vi "Send Message.vi"(0 "object in":refnum<class "Laser_Ethernet.lvclass">, 5 "error in (no error)":errorcluster) -> (14 "object out":refnum<class "Laser_Ethernet.lvclass">, 19 "error out":errorcluster)   [LabVIEW 2023, in "Laser_Ethernet.lvclass"]
uses:
  Laser_Ethernet.lvclass
  Laser_Ethernet.lvclass/Laser_Ethernet.ctl
panel:
  in  "Size of Data":u32
  in  "Command":u16
  in  "Data":variant
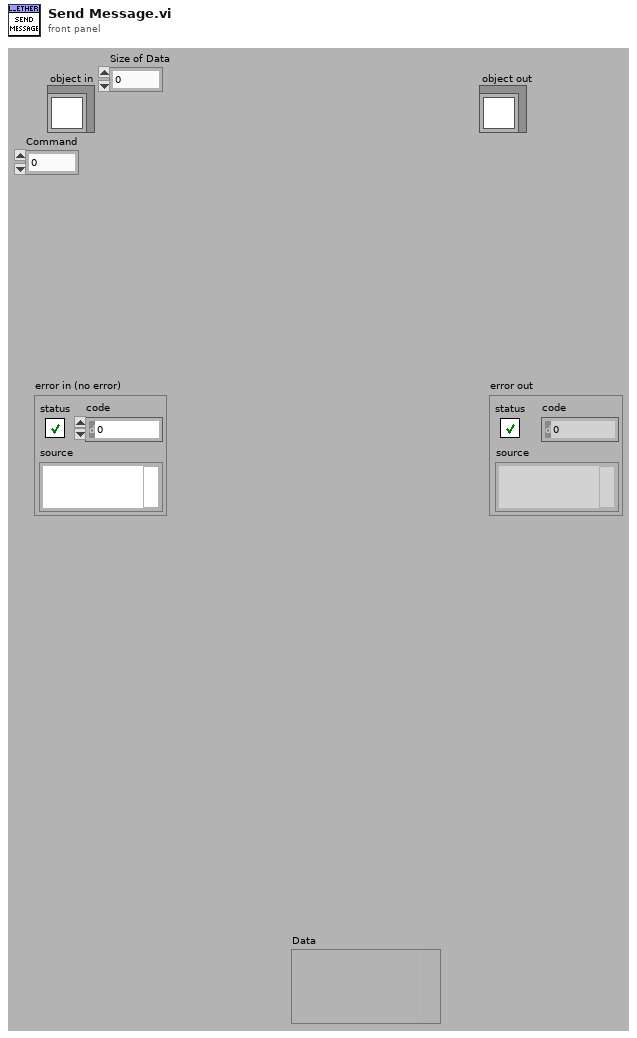
[diagram p1: front panel]
types:
  T1 = enum16{"big-endian, network order", "native, host order", "little-endian"}
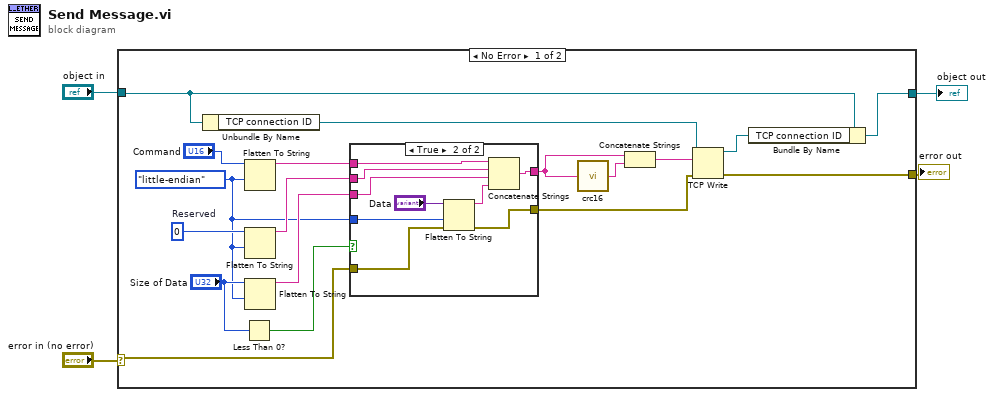
[diagram p0: block diagram]
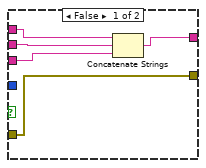
[diagram p2: hidden frame]
diagram:
  n1 = case shown="No Error" "error in (no error)" {
    selector: "error in (no error)" -> [w13 w38]
    tunnel: [w11 w38] -> w3
    tunnel: [w10 w37] -> w1
    tunnel: "object in" -> [w8 w37]
    frame No Error {
      w20 = u16 0  # Reserved
      w14 = T1."little-endian" ("byte order (0:big-endian, network order)")
      n2 = Unbundle By Name(w8) -> ("TCP connection ID"=w12:refnum<k5>)
      n3 = Less Than 0?(x="Size of Data") -> (x < 0?=w15:bool)
      n4 = Flatten To String(anything="Command", byte order (0:big-endian, network order)=w14) -> (data string=w21:string)  [unwired: 2 in, 2 out]
      n5 = Flatten To String(anything=w20, byte order (0:big-endian, network order)=w14) -> (data string=w19:string)  [unwired: 2 in, 2 out]
      n6 = Flatten To String(anything="Size of Data", byte order (0:big-endian, network order)=w14) -> (data string=w18:string)  [unwired: 2 in, 2 out]
      n7 = case shown="True" w15 {
        tunnel: w21 -> [w27 w36]
        tunnel: w19 -> [w25 w35]
        tunnel: w18 -> [w24 w34]
        tunnel: [w26 w33] -> w7
        tunnel: w14 -> [_ w31]
        tunnel: w13 -> [w23 w29]
        tunnel: [w23 w28] -> w5
        frame False {
          n8 = Concatenate Strings(w27, w25, w24) -> (w26:string)
        }
        frame True {
          n9 = Flatten To String(anything="Data", byte order (0:big-endian, network order)=w31, error in (no error)=w29) -> (data string=w32:string, error out=w28:errorcluster)  [unwired: 1 in, 1 out]
          n10 = Concatenate Strings(w36, w35, w34, w32) -> (w33:string)
        }
      }
      n11 = call "crc16.vi"("Message"=w7) -> ("crc 16"=w6:string)
      n12 = Concatenate Strings(w7, w6) -> (w17:string)
      n13 = TCP Write(connection ID=w12, data in=w17, error in (no error)=w5) -> (connection ID out=w9:refnum<k5>, error out=w11:errorcluster)  [unwired: 1 in, 1 out]
      n14 = Bundle By Name(cluster=w8, "TCP connection ID"=w9) -> (w10:refnum<class "Laser_Ethernet.lvclass">)
    }
    frame Error {
    }
  }
  "error out" <- w3
  "object out" <- w1
